vi "save tiff under file path.vi"(8 "error in (no error)":errorcluster, 9 "tiff name":string, 10 "Image":T1, 11 "Thorcam in":refnum<class "Thorcam.lvclass">) -> (0 "error out":errorcluster, 3 "Thorcam out":refnum<class "Thorcam.lvclass">)   [LabVIEW 2012, in "Thorcam.lvclass"]
uses:
  Thorcam.lvclass
  <vilib>/vision/Image Controls.llb/IMAQ Image.ctl
  Thorcam.lvclass/Thorcam.ctl
  <vilib>/vision/NI_Vision_Development_Module.lvlib
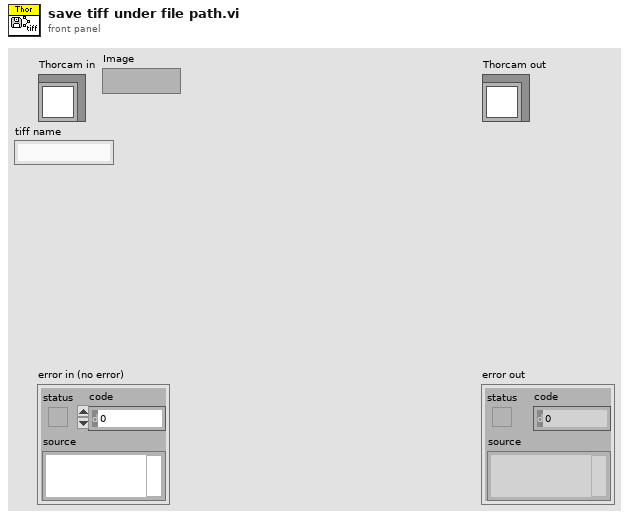
[diagram p1: front panel]
types:
  T1 = typedef "IMAQ Image.ctl" = refnum<image>
  T2 = cluster{"Rows Per Strip":i32, "Photometric":i32, "Compression Type":i32}
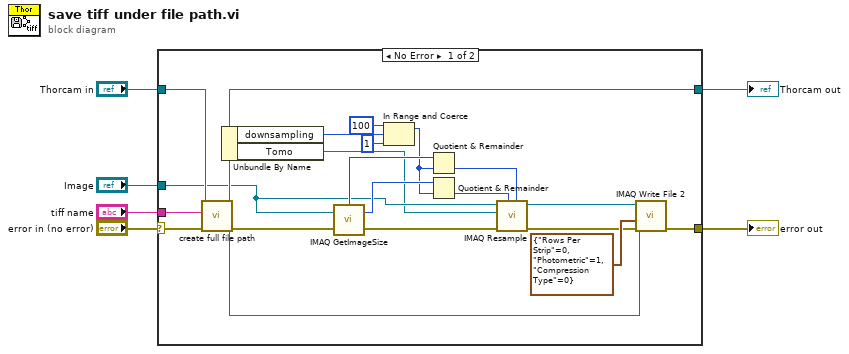
[diagram p0: block diagram]
diagram:
  n1 = case shown="No Error" "error in (no error)" {
    selector: "error in (no error)" -> [w26 w29]
    tunnel: [w24 w29] -> w5
    tunnel: [w14 w28] -> w3
    tunnel: "Thorcam in" -> [w27 w28]
    tunnel: "tiff name" -> [w25 _]
    tunnel: "Image" -> [w10 _]
    frame No Error {
      n2 = call-dynamic "create full file path.vi"("error in (no error)"=w26, "String"=w25, "Thorcam in"=w27) -> ("error out"=w12:errorcluster, "full file path"=w22:path, "Thorcam out"=w14:refnum<class "Thorcam.lvclass">)  [unwired: 6 in]
      n3 = Unbundle By Name(w14) -> ("downsampling"=w9:i32, "Tomo"=w8:T1)
      n4 = call "IMAQ GetImageSize"("Image"=w10, "error in (no error)"=w12) -> ("Y Resolution"=w20:i32, "X Resolution"=w21:i32, "error out"=w13:errorcluster)  [unwired: 2 in]
      n5 = In Range and Coerce(upper limit=100, x=w9, lower limit=1 ("upper limit")) -> (coerced(x)=w19:i32)  [unwired: 1 out]
      n6 = Quotient & Remainder(x=w21, y=w19) -> (floor(x/y)=w17:i32)  [unwired: 1 out]
      n7 = Quotient & Remainder(x=w20, y=w19) -> (floor(x/y)=w18:i32)  [unwired: 1 out]
      n8 = call "IMAQ Resample"("X Resolution"=w17, "Y Resolution"=w18, "error in (no error)"=w13, "Image Dst"=w8, "Image Src"=w10) -> ("error out"=w11:errorcluster, "Image Dst Out"=w7:T1)  [unwired: 5 in]
      n9 = call-poly "IMAQ Write File 2"("error in (no error)"=w11, "TIFF Options"=T2 {"Rows Per Strip"=0, "Photometric"=1, "Compression Type"=0}, "File Path"=w22, "Image"=w7) -> ("error out"=w24:errorcluster)  [unwired: 6 in, 1 out]
    }
    frame Error {
    }
  }
  "error out" <- w5
  "Thorcam out" <- w3
